vi "Introduce.vi"(8 "Error In":errorcluster, 11 "BB-Series in":refnum<class "BB-Series.lvclass">) -> (0 "Error Out":errorcluster, 3 "BB-Series out":refnum<class "BB-Series.lvclass">)   [LabVIEW 2021, in "BB-Series.lvclass"]
doc: "Show ID of droid in prompt message for user. Comments in Polish."
uses:
  BB-Series.lvclass
  BB-Series.lvclass/BB-Series.ctl
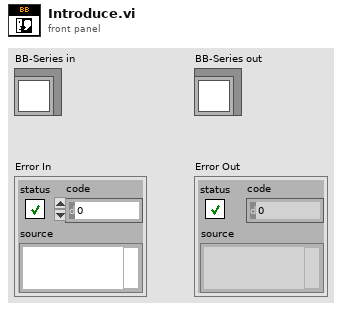
[diagram p1: front panel]
types:
  T1 = enum16{"Q-Series", "BB-Series", "C-Series", "R-Series"}
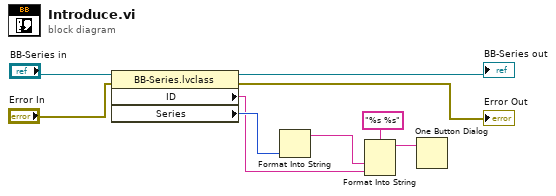
[diagram p0: block diagram]
diagram:
  n1 = property class="BB-Series.lvclass"(reference="BB-Series in", error in="Error In") -> (reference out=→"BB-Series out":refnum<class "BB-Series.lvclass">, error out=→"Error Out":errorcluster, "ID"=w2:string, "Series"=w5:T1)
  n2 = Format Into String(w5) -> (resulting string=w3:string)  [unwired: 3 in, 1 out]
  n3 = Format Into String(format string="%s %s", w3, w2) -> (resulting string=w1:string)  [unwired: 2 in, 1 out]
  n4 = One Button Dialog(message=w1) -> ()  [unwired: 1 in, 1 out]
